vi "CentralStorage.RequestVar.vi"(8 "Error In":errorcluster, 10 "Variant":variant, 11 "CentralStorage (optional)":refnum<data-value>) -> (0 "Error Out":errorcluster, 2 "VariantRef":refnum<data-value>, 3 "CentralStorage":refnum<data-value>)   [LabVIEW 2016, in "CentralStorage.lvclass"]
uses:
  CentralStorage.lvclass
  CentralStorage.ReferenceRequest.ctl
  CentralStorage.DataTypes.ctl
  CentralStorage.lvclass/CentralStorage.ctl
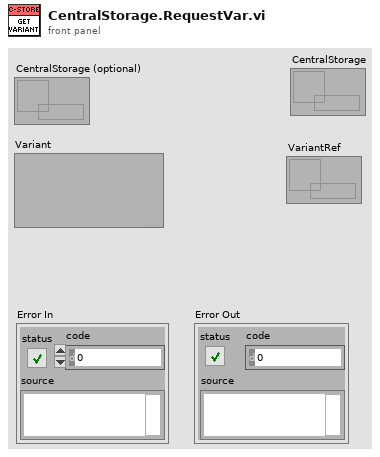
[diagram p1: front panel]
types:
  T1 = typedef "CentralStorage.lvclass/CentralStorage.DataTypes.ctl" = enum16{"Variant Array", "Variant", "Waveform"}
  T2 = typedef "CentralStorage.lvclass/CentralStorage.ReferenceRequest.ctl" = cluster{"Caller":string, "DataType":T1, "Data":variant}
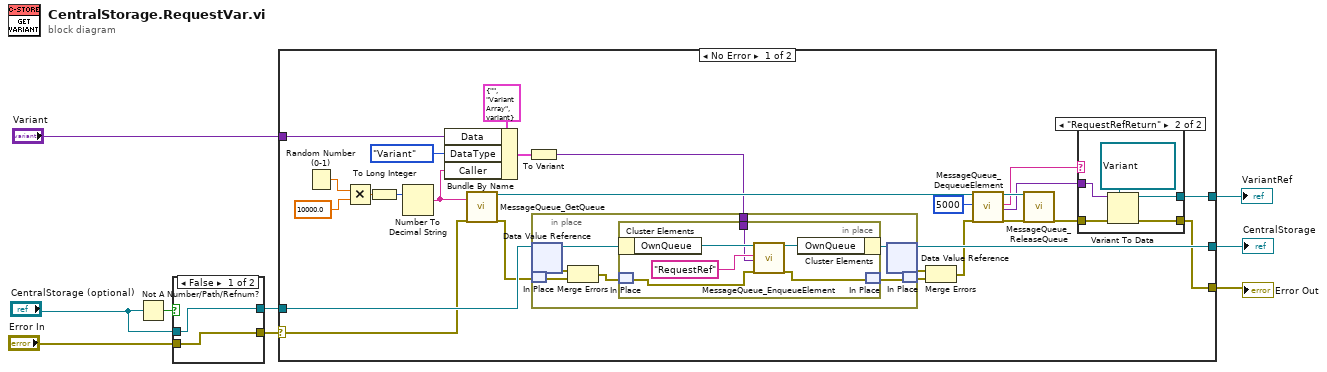
[diagram p0: block diagram]
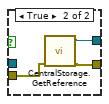
[diagram p2: hidden frame]
diagram:
  n1 = Not A Number/Path/Refnum?(number/path/refnum="CentralStorage (optional)") -> (NaN/Path/Refnum?=w7:bool)
  n2 = case shown="False" w7 {
    tunnel: "CentralStorage (optional)" -> [w11 _]
    tunnel: "Error In" -> [w10 w14]
    tunnel: [w11 w12] -> w4
    tunnel: [w10 w13] -> w8
    frame False {
    }
    frame True {
      n3 = call "CentralStorage.GetReference.vi"("Error in"=w14) -> ("Error out"=w13:errorcluster, "CentralStorage"=w12:refnum<data-value>)  [unwired: 9 in]
    }
  }
  n4 = case shown="No Error" w8 {
    selector: w8 -> [w28 w61]
    tunnel: [w17 w61] -> w9
    tunnel: w4 -> [w40 w60]
    tunnel: [w39 w60] -> w3
    tunnel: "Variant" -> [w32 _]
    tunnel: [w16 _] -> w1
    frame No Error {
      n5 = Random Number (0-1)() -> (number: 0 to 1=w36:dbl)
      n6 = Multiply(x=w36, y=10000.0) -> (x*y=w37:dbl)
      n7 = To Long Integer(number=w37) -> (32bit integer=w38:i32)
      n8 = Number To Decimal String(number=w38) -> (decimal integer string=w29:string)  [unwired: 1 in]
      n9 = Bundle By Name(cluster=T2 {"Caller"="", "DataType"=enum."Variant Array", "Data"=variant} ("ReferenceRequest"), "Data"=w32, "DataType"=CentralStorage.DataTypes."Variant", "Caller"=w29) -> (w26:T2)
      n10 = call "MessageQueue_GetQueue.vi"("Name"=w29, "ErrorIn"=w28) -> ("QueueOut"=w22:refnum<queue>, "ErrorOut"=w27:errorcluster)  [unwired: 15 in, 1 out]
      n11 = To Variant(anything=w26) -> (Variant=w15:variant)
      n12 = in-place {
        in-place-border: w15 -> [w47]
        n13 = in-place-dvr #1(w40) -> (w53:refnum<class "CentralStorage.lvclass">, w51:errorcluster)
        n14 = in-place-match #2(w27) -> (w50:errorcluster)
        n15 = Merge Errors(w51, w50) -> (w49:errorcluster)
        n16 = in-place {
          in-place-border: w47 -> [w54]
          n17 = in-place-cluster #3(w53) -> ("OwnQueue"=w59:refnum<queue>)
          n18 = in-place-match #4(w49) -> (w56:errorcluster)
          n19 = call "MessageQueue_EnqueueElement.vi"("QueueIn"=w59, "Message"="RequestRef", "Data"=w54, "ErrorIn"=w56) -> ("QueueOut"=w58:refnum<queue>, "ErrorOut"=w55:errorcluster)  [unwired: 14 in]
          n20 = in-place-cluster #3("OwnQueue"=w58) -> (w52:refnum<class "CentralStorage.lvclass">)
          n21 = in-place-match #4(w55) -> (w48:errorcluster)
        }
        n22 = in-place-dvr #1(w52) -> (w39:refnum<data-value>, w30:errorcluster)
        n23 = in-place-match #2(w48) -> (w31:errorcluster)
      }
      n24 = Merge Errors(w30, w31) -> (w25:errorcluster)
      n25 = call "MessageQueue_DequeueElement.vi"("QueueIn"=w22, "Timeout"=5000, "ErrorIn"=w25) -> ("QueueOut"=w23:refnum<queue>, "Message"=w20:string, "Data"=w19:variant, "ErrorOut"=w24:errorcluster)  [unwired: 12 in, 1 out]
      n26 = call "MessageQueue_ReleaseQueue.vi"("QueueIn"=w23, "ErrorIn"=w24) -> ("ErrorOut"=w18:errorcluster)  [unwired: 15 in, 2 out]
      n27 = case shown="\"RequestRefReturn\"" w20 {
        tunnel: w19 -> [_ w44]
        tunnel: w18 -> [w41 w46]
        tunnel: [w41 w45] -> w17
        tunnel: [_ w43] -> w16
        frame Default {
        }
        frame "RequestRefReturn" {
          n28 = Variant To Data(error in=w46, type=refnum<data-value> refnum ("data value reference"), Variant=w44) -> (data=w43:refnum<data-value>, error out=w45:errorcluster)
        }
      }
    }
    frame Error {
    }
  }
  "Error Out" <- w9
  "CentralStorage" <- w3
  "VariantRef" <- w1
